vi "Resample (constant to variable).vi"   [LabVIEW 2017, in "NI_AALPro.lvlib"]
doc: "Resamples input signal <B>X</B> according to <B>Time</B> using an FIR filter implementation. Wire data to the <B>X</B> input to determine the polymorphic instance to use or manually select the instance."
uses:
  <vilib>/Analysis/NI_AALPro.lvlib
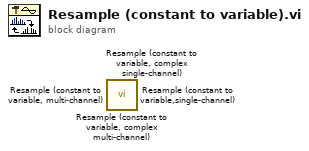
[diagram p0: block diagram]
diagram:
  n1 = call <vilib>:"Resample (constant to variable, complex multi-channel).vi"() -> ()  [unwired: 9 in, 3 out]
  n2 = call <vilib>:"Resample (constant to variable, complex single-channel).vi"() -> ()  [unwired: 9 in, 3 out]
  n3 = call <vilib>:"Resample (constant to variable, multi-channel).vi"() -> ()  [unwired: 9 in, 3 out]
  n4 = call <vilib>:"Resample (constant to variable,single-channel).vi"() -> ()  [unwired: 9 in, 3 out]
